vi "CFG Convert String to VISA.vi"(5 "VISA String":string) -> (2 "VISA Resource":refnum<visa-resource-name>)   [LabVIEW 2012]
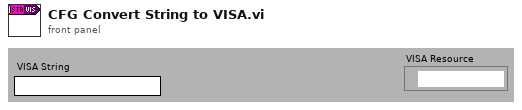
[diagram p1: front panel]
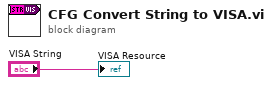
[diagram p0: block diagram]
diagram:
  "VISA Resource" <- "VISA String"
